vi "Shock&Dyanamics Laboratory - DROPBEAR_June2022_Rev3.vi"() -> ()   [LabVIEW 2019] (continued)
                n641 = property on="Sensitivity 20" class="DigNum (strict)"(error in=w164, "DisabledEnum"=w160) -> (error out=w163:errorcluster)  [unwired: 1 in, 1 out]
                n642 = property on="Sensitivity 19" class="DigNum (strict)"(error in=w173, "DisabledEnum"=w177) -> (error out=w174:errorcluster)  [unwired: 1 in, 1 out]
                n643 = property on="Name Ch 1" class="Str"(error in=w371, "DisabledEnum"=w365) -> (error out=w370:errorcluster)  [unwired: 1 in, 1 out]
                n644 = property on="Physical Channel Ch 27" class="DAQmxName"(error in=w104, "DisabledEnum"=w97) -> (error out=w103:errorcluster)  [unwired: 1 in, 1 out]
                n645 = property on="Name Ch 2" class="Str"(error in=w362, "DisabledEnum"=w356) -> (error out=w361:errorcluster)  [unwired: 1 in, 1 out]
                n646 = property on="Name Ch 4" class="Str"(error in=w346, "DisabledEnum"=w340) -> (error out=w345:errorcluster)  [unwired: 1 in, 1 out]
                n647 = property on="Name Ch 5" class="Str"(error in=w331, "DisabledEnum"=w325) -> (error out=w330:errorcluster)  [unwired: 1 in, 1 out]
                n648 = property on="Name Ch 6" class="Str"(error in=w321, "DisabledEnum"=w315) -> (error out=w320:errorcluster)  [unwired: 1 in, 1 out]
                n649 = property on="Name Ch 12" class="Str"(error in=w262, "DisabledEnum"=w256) -> (error out=w261:errorcluster)  [unwired: 1 in, 1 out]
                n650 = property on="Name Ch 13" class="Str"(error in=w253, "DisabledEnum"=w247) -> (error out=w252:errorcluster)  [unwired: 1 in, 1 out]
                n651 = property on="Name Ch 15" class="Str"(error in=w235, "DisabledEnum"=w229) -> (error out=w234:errorcluster)  [unwired: 1 in, 1 out]
                n652 = property on="Name Ch 7" class="Str"(error in=w312, "DisabledEnum"=w306) -> (error out=w311:errorcluster)  [unwired: 1 in, 1 out]
                n653 = property on="Name Ch 11" class="Str"(error in=w271, "DisabledEnum"=w265) -> (error out=w270:errorcluster)  [unwired: 1 in, 1 out]
                n654 = property on="Name Ch 14" class="Str"(error in=w244, "DisabledEnum"=w238) -> (error out=w243:errorcluster)  [unwired: 1 in, 1 out]
                n655 = property on="Name Ch 8" class="Str"(error in=w301, "DisabledEnum"=w295) -> (error out=w300:errorcluster)  [unwired: 1 in, 1 out]
                n656 = property on="Name Ch 9" class="Str"(error in=w292, "DisabledEnum"=w286) -> (error out=w291:errorcluster)  [unwired: 1 in, 1 out]
                n657 = property on="Name Ch 10" class="Str"(error in=w283, "DisabledEnum"=w277) -> (error out=w282:errorcluster)  [unwired: 1 in, 1 out]
                n658 = property on="Name Ch 16" class="Str"(error in=w220, "DisabledEnum"=w197) -> (error out=w219:errorcluster)  [unwired: 1 in, 1 out]
                n659 = property on="PF Condition 24" class="Bool (strict)"(error in=w130, "DisabledEnum"=w124) -> (error out=w129:errorcluster)  [unwired: 1 in, 1 out]
                n660 = property on="Name Ch 3" class="Str"(error in=w354, "DisabledEnum"=w348) -> (error out=w353:errorcluster)  [unwired: 1 in, 1 out]
                n661 = property on="PF Condition 23" class="Bool (strict)"(error in=w138, "DisabledEnum"=w125) -> (error out=w137:errorcluster)  [unwired: 1 in, 1 out]
                n662 = property on="PF Condition 22" class="Bool (strict)"(error in=w146, "DisabledEnum"=w126) -> (error out=w145:errorcluster)  [unwired: 1 in, 1 out]
                n663 = property on="PF Condition 21" class="Bool (strict)"(error in=w154, "DisabledEnum"=w127) -> (error out=w153:errorcluster)  [unwired: 1 in, 1 out]
                n664 = property on="Sens Fac 17" class="Enum (strict)"(error in=w192, "DisabledEnum"=w187) -> (error out=w188:errorcluster)  [unwired: 1 in, 1 out]
                n665 = property on="PF Condition 20" class="Bool (strict)"(error in=w163, "DisabledEnum"=w160) -> (error out=w162:errorcluster)  [unwired: 1 in, 1 out]
                n666 = property on="PF Condition 19" class="Bool (strict)"(error in=w174, "DisabledEnum"=w177) -> (error out=w175:errorcluster)  [unwired: 1 in, 1 out]
                n667 = property on="PF Condition 18" class="Bool (strict)"(error in=w181, "DisabledEnum"=w178) -> (error out=w180:errorcluster)  [unwired: 1 in, 1 out]
                n668 = property on="Sens Fac 1" class="Enum (strict)"(error in=w370, "DisabledEnum"=w365) -> (error out=w369:errorcluster)  [unwired: 1 in, 1 out]
                n669 = property on="Sens Fac 2" class="Enum (strict)"(error in=w361, "DisabledEnum"=w356) -> (error out=w360:errorcluster)  [unwired: 1 in, 1 out]
                n670 = property on="Name Ch 30" class="Str"(error in=w72, "DisabledEnum"=w78) -> (error out=w73:errorcluster)  [unwired: 1 in, 1 out]
                n671 = property on="Sens Fac 4" class="Enum (strict)"(error in=w345, "DisabledEnum"=w340) -> (error out=w344:errorcluster)  [unwired: 1 in, 1 out]
                n672 = property on="Sens Fac 5" class="Enum (strict)"(error in=w330, "DisabledEnum"=w325) -> (error out=w329:errorcluster)  [unwired: 1 in, 1 out]
                n673 = property on="Sens Fac 6" class="Enum (strict)"(error in=w320, "DisabledEnum"=w315) -> (error out=w319:errorcluster)  [unwired: 1 in, 1 out]
                n674 = property on="Sens Fac 12" class="Enum (strict)"(error in=w261, "DisabledEnum"=w256) -> (error out=w260:errorcluster)  [unwired: 1 in, 1 out]
                n675 = property on="Sens Fac 13" class="Enum (strict)"(error in=w252, "DisabledEnum"=w247) -> (error out=w251:errorcluster)  [unwired: 1 in, 1 out]
                n676 = property on="Sens Fac 15" class="Enum (strict)"(error in=w234, "DisabledEnum"=w229) -> (error out=w233:errorcluster)  [unwired: 1 in, 1 out]
                n677 = property on="Sens Fac 7" class="Enum (strict)"(error in=w311, "DisabledEnum"=w306) -> (error out=w310:errorcluster)  [unwired: 1 in, 1 out]
                n678 = property on="Sens Fac 11" class="Enum (strict)"(error in=w270, "DisabledEnum"=w265) -> (error out=w269:errorcluster)  [unwired: 1 in, 1 out]
                n679 = property on="Sens Fac 14" class="Enum (strict)"(error in=w243, "DisabledEnum"=w238) -> (error out=w242:errorcluster)  [unwired: 1 in, 1 out]
                n680 = property on="Sens Fac 8" class="Enum (strict)"(error in=w300, "DisabledEnum"=w295) -> (error out=w299:errorcluster)  [unwired: 1 in, 1 out]
                n681 = property on="Sens Fac 9" class="Enum (strict)"(error in=w291, "DisabledEnum"=w286) -> (error out=w290:errorcluster)  [unwired: 1 in, 1 out]
                n682 = property on="Sens Fac 10" class="Enum (strict)"(error in=w282, "DisabledEnum"=w277) -> (error out=w281:errorcluster)  [unwired: 1 in, 1 out]
                n683 = property on="Sens Fac 16" class="Enum (strict)"(error in=w219, "DisabledEnum"=w197) -> (error out=w218:errorcluster)  [unwired: 1 in, 1 out]
                n684 = property on="Name Ch 29" class="Str"(error in=w81, "DisabledEnum"=w87) -> (error out=w82:errorcluster)  [unwired: 1 in, 1 out]
                n685 = property on="Name Ch 25" class="Str"(error in=w121, "DisabledEnum"=w115) -> (error out=w120:errorcluster)  [unwired: 1 in, 1 out]
                n686 = property on="Name Ch 26" class="Str"(error in=w108, "DisabledEnum"=w114) -> (error out=w109:errorcluster)  [unwired: 1 in, 1 out]
                n687 = property on="Sens Fac 3" class="Enum (strict)"(error in=w353, "DisabledEnum"=w348) -> (error out=w352:errorcluster)  [unwired: 1 in, 1 out]
                n688 = property on="Name Ch 28" class="Str"(error in=w90, "DisabledEnum"=w96) -> (error out=w91:errorcluster)  [unwired: 1 in, 1 out]
                n689 = property on="Name Ch 27" class="Str"(error in=w103, "DisabledEnum"=w97) -> (error out=w102:errorcluster)  [unwired: 1 in, 1 out]
                n690 = property on="Name Ch 31" class="Str"(error in=w63, "DisabledEnum"=w69) -> (error out=w64:errorcluster)  [unwired: 1 in, 1 out]
                n691 = property on="Sensitivity 17" class="DigNum (strict)"(error in=w188, "DisabledEnum"=w187) -> (error out=w189:errorcluster)  [unwired: 1 in, 1 out]
                n692 = property on="Voltage Min Ch 24" class="DigNum (strict)"(error in=w129, "DisabledEnum"=w124) -> (error out=w128:errorcluster)  [unwired: 1 in, 1 out]
                n693 = property on="Voltage Min Ch 23" class="DigNum (strict)"(error in=w137, "DisabledEnum"=w125) -> (error out=w136:errorcluster)  [unwired: 1 in, 1 out]
                n694 = property on="Sensitivity 1" class="DigNum (strict)"(error in=w369, "DisabledEnum"=w365) -> (error out=w368:errorcluster)  [unwired: 1 in, 1 out]
                n695 = property on="Voltage Min Ch 21" class="DigNum (strict)"(error in=w153, "DisabledEnum"=w127) -> (error out=w152:errorcluster)  [unwired: 1 in, 1 out]
                n696 = property on="Voltage Min Ch 22" class="DigNum (strict)"(error in=w145, "DisabledEnum"=w126) -> (error out=w144:errorcluster)  [unwired: 1 in, 1 out]
                n697 = property on="Voltage Min Ch 20" class="DigNum (strict)"(error in=w162, "DisabledEnum"=w160) -> (error out=w161:errorcluster)  [unwired: 1 in, 1 out]
                n698 = property on="Voltage Min Ch 18" class="DigNum (strict)"(error in=w180, "DisabledEnum"=w178) -> (error out=w179:errorcluster)  [unwired: 1 in, 1 out]
                n699 = property on="Voltage Min Ch 19" class="DigNum (strict)"(error in=w175, "DisabledEnum"=w177) -> (error out=w176:errorcluster)  [unwired: 1 in, 1 out]
                n700 = property on="Sensitivity 2" class="DigNum (strict)"(error in=w360, "DisabledEnum"=w356) -> (error out=w359:errorcluster)  [unwired: 1 in, 1 out]
                n701 = property on="Sensitivity 4" class="DigNum (strict)"(error in=w344, "DisabledEnum"=w340) -> (error out=w343:errorcluster)  [unwired: 1 in, 1 out]
                n702 = property on="Sensitivity 5" class="DigNum (strict)"(error in=w329, "DisabledEnum"=w325) -> (error out=w328:errorcluster)  [unwired: 1 in, 1 out]
                n703 = property on="Sensitivity 6" class="DigNum (strict)"(error in=w319, "DisabledEnum"=w315) -> (error out=w318:errorcluster)  [unwired: 1 in, 1 out]
                n704 = property on="Sensitivity 12" class="DigNum (strict)"(error in=w260, "DisabledEnum"=w256) -> (error out=w259:errorcluster)  [unwired: 1 in, 1 out]
                n705 = property on="Sensitivity 13" class="DigNum (strict)"(error in=w251, "DisabledEnum"=w247) -> (error out=w250:errorcluster)  [unwired: 1 in, 1 out]
                n706 = property on="Sensitivity 15" class="DigNum (strict)"(error in=w233, "DisabledEnum"=w229) -> (error out=w232:errorcluster)  [unwired: 1 in, 1 out]
                n707 = property on="Sensitivity 7" class="DigNum (strict)"(error in=w310, "DisabledEnum"=w306) -> (error out=w309:errorcluster)  [unwired: 1 in, 1 out]
                n708 = property on="Sensitivity 11" class="DigNum (strict)"(error in=w269, "DisabledEnum"=w265) -> (error out=w268:errorcluster)  [unwired: 1 in, 1 out]
                n709 = property on="Sensitivity 14" class="DigNum (strict)"(error in=w242, "DisabledEnum"=w238) -> (error out=w241:errorcluster)  [unwired: 1 in, 1 out]
                n710 = property on="Sensitivity 8" class="DigNum (strict)"(error in=w299, "DisabledEnum"=w295) -> (error out=w298:errorcluster)  [unwired: 1 in, 1 out]
                n711 = property on="Sensitivity 9" class="DigNum (strict)"(error in=w290, "DisabledEnum"=w286) -> (error out=w289:errorcluster)  [unwired: 1 in, 1 out]
                n712 = property on="Sensitivity 10" class="DigNum (strict)"(error in=w281, "DisabledEnum"=w277) -> (error out=w280:errorcluster)  [unwired: 1 in, 1 out]
                n713 = property on="Sensitivity 16" class="DigNum (strict)"(error in=w218, "DisabledEnum"=w197) -> (error out=w217:errorcluster)  [unwired: 1 in, 1 out]
                n714 = property on="Sensitivity 3" class="DigNum (strict)"(error in=w352, "DisabledEnum"=w348) -> (error out=w351:errorcluster)  [unwired: 1 in, 1 out]
                n715 = property on="Sens Fac 30" class="Enum (strict)"(error in=w73, "DisabledEnum"=w78) -> (error out=w74:errorcluster)  [unwired: 1 in, 1 out]
                n716 = property on="Sens Fac 27" class="Enum (strict)"(error in=w102, "DisabledEnum"=w97) -> (error out=w101:errorcluster)  [unwired: 1 in, 1 out]
                n717 = property on="Sens Fac 29" class="Enum (strict)"(error in=w82, "DisabledEnum"=w87) -> (error out=w83:errorcluster)  [unwired: 1 in, 1 out]
                n718 = property on="PF Condition 17" class="Bool (strict)"(error in=w189, "DisabledEnum"=w187) -> (error out=w190:errorcluster)  [unwired: 1 in, 1 out]
                n719 = property on="Sens Fac 26" class="Enum (strict)"(error in=w109, "DisabledEnum"=w114) -> (error out=w110:errorcluster)  [unwired: 1 in, 1 out]
                n720 = property on="Sens Fac 25" class="Enum (strict)"(error in=w120, "DisabledEnum"=w115) -> (error out=w119:errorcluster)  [unwired: 1 in, 1 out]
                n721 = property on="Sens Fac 28" class="Enum (strict)"(error in=w91, "DisabledEnum"=w96) -> (error out=w92:errorcluster)  [unwired: 1 in, 1 out]
                n722 = property on="PF Condition 1" class="Bool (strict)"(error in=w368, "DisabledEnum"=w365) -> (error out=w364:errorcluster)  [unwired: 1 in, 1 out]
                n723 = property on="PF Condition 2" class="Bool (strict)"(error in=w359, "DisabledEnum"=w356) -> (error out=w355:errorcluster)  [unwired: 1 in, 1 out]
                n724 = property on="PF Condition 4" class="Bool (strict)"(error in=w343, "DisabledEnum"=w340) -> (error out=w339:errorcluster)  [unwired: 1 in, 1 out]
                n725 = property on="PF Condition 5" class="Bool (strict)"(error in=w328, "DisabledEnum"=w325) -> (error out=w324:errorcluster)  [unwired: 1 in, 1 out]
                n726 = property on="PF Condition 6" class="Bool (strict)"(error in=w318, "DisabledEnum"=w315) -> (error out=w314:errorcluster)  [unwired: 1 in, 1 out]
                n727 = property on="PF Condition 12" class="Bool (strict)"(error in=w259, "DisabledEnum"=w256) -> (error out=w255:errorcluster)  [unwired: 1 in, 1 out]
                n728 = property on="PF Condition 13" class="Bool (strict)"(error in=w250, "DisabledEnum"=w247) -> (error out=w246:errorcluster)  [unwired: 1 in, 1 out]
                n729 = property on="PF Condition 15" class="Bool (strict)"(error in=w232, "DisabledEnum"=w229) -> (error out=w228:errorcluster)  [unwired: 1 in, 1 out]
                n730 = property on="Sens Fac 31" class="Enum (strict)"(error in=w64, "DisabledEnum"=w69) -> (error out=w65:errorcluster)  [unwired: 1 in, 1 out]
                n731 = property on="PF Condition 7" class="Bool (strict)"(error in=w309, "DisabledEnum"=w306) -> (error out=w305:errorcluster)  [unwired: 1 in, 1 out]
                n732 = property on="PF Condition 11" class="Bool (strict)"(error in=w268, "DisabledEnum"=w265) -> (error out=w264:errorcluster)  [unwired: 1 in, 1 out]
                n733 = property on="PF Condition 14" class="Bool (strict)"(error in=w241, "DisabledEnum"=w238) -> (error out=w237:errorcluster)  [unwired: 1 in, 1 out]
                n734 = property on="PF Condition 8" class="Bool (strict)"(error in=w298, "DisabledEnum"=w295) -> (error out=w294:errorcluster)  [unwired: 1 in, 1 out]
                n735 = property on="PF Condition 9" class="Bool (strict)"(error in=w289, "DisabledEnum"=w286) -> (error out=w285:errorcluster)  [unwired: 1 in, 1 out]
                n736 = property on="PF Condition 10" class="Bool (strict)"(error in=w280, "DisabledEnum"=w277) -> (error out=w276:errorcluster)  [unwired: 1 in, 1 out]
                n737 = property on="Voltage Max Ch 24" class="DigNum (strict)"(error in=w128, "DisabledEnum"=w124) -> ()  [unwired: 1 in, 2 out]
                n738 = property on="PF Condition 16" class="Bool (strict)"(error in=w217, "DisabledEnum"=w197) -> (error out=w215:errorcluster)  [unwired: 1 in, 1 out]
                n739 = property on="Voltage Max Ch 23" class="DigNum (strict)"(error in=w136, "DisabledEnum"=w125) -> ()  [unwired: 1 in, 2 out]
                n740 = property on="Voltage Max Ch 19" class="DigNum (strict)"(error in=w176, "DisabledEnum"=w177) -> ()  [unwired: 1 in, 2 out]
                n741 = property on="Voltage Max Ch 21" class="DigNum (strict)"(error in=w152, "DisabledEnum"=w127) -> ()  [unwired: 1 in, 2 out]
                n742 = property on="Voltage Max Ch 18" class="DigNum (strict)"(error in=w179, "DisabledEnum"=w178) -> ()  [unwired: 1 in, 2 out]
                n743 = property on="PF Condition 3" class="Bool (strict)"(error in=w351, "DisabledEnum"=w348) -> (error out=w347:errorcluster)  [unwired: 1 in, 1 out]
                n744 = property on="Voltage Max Ch 20" class="DigNum (strict)"(error in=w161, "DisabledEnum"=w160) -> ()  [unwired: 1 in, 2 out]
                n745 = property on="Voltage Max Ch 22" class="DigNum (strict)"(error in=w144, "DisabledEnum"=w126) -> ()  [unwired: 1 in, 2 out]
                n746 = property on="Sensitivity 28" class="DigNum (strict)"(error in=w92, "DisabledEnum"=w96) -> (error out=w93:errorcluster)  [unwired: 1 in, 1 out]
                n747 = property on="Sensitivity 30" class="DigNum (strict)"(error in=w74, "DisabledEnum"=w78) -> (error out=w75:errorcluster)  [unwired: 1 in, 1 out]
                n748 = property on="Sensitivity 25" class="DigNum (strict)"(error in=w119, "DisabledEnum"=w115) -> (error out=w118:errorcluster)  [unwired: 1 in, 1 out]
                n749 = property on="Sensitivity 29" class="DigNum (strict)"(error in=w83, "DisabledEnum"=w87) -> (error out=w84:errorcluster)  [unwired: 1 in, 1 out]
                n750 = property on="Sensitivity 26" class="DigNum (strict)"(error in=w110, "DisabledEnum"=w114) -> (error out=w111:errorcluster)  [unwired: 1 in, 1 out]
                n751 = property on="Sensitivity 27" class="DigNum (strict)"(error in=w101, "DisabledEnum"=w97) -> (error out=w100:errorcluster)  [unwired: 1 in, 1 out]
                n752 = property on="Voltage Max Ch 1" class="DigNum (strict)"(error in=w364, "DisabledEnum"=w365) -> (error out=w366:errorcluster)  [unwired: 1 in, 1 out]
                n753 = property on="Voltage Max Ch 17" class="DigNum (strict)"(error in=w190, "DisabledEnum"=w187) -> (error out=w191:errorcluster)  [unwired: 1 in, 1 out]
                n754 = property on="Sensitivity 31" class="DigNum (strict)"(error in=w65, "DisabledEnum"=w69) -> (error out=w66:errorcluster)  [unwired: 1 in, 1 out]
                n755 = property on="Voltage Max Ch 2" class="DigNum (strict)"(error in=w355, "DisabledEnum"=w356) -> (error out=w357:errorcluster)  [unwired: 1 in, 1 out]
                n756 = property on="Voltage Max Ch 4" class="DigNum (strict)"(error in=w339, "DisabledEnum"=w340) -> (error out=w341:errorcluster)  [unwired: 1 in, 1 out]
                n757 = property on="Voltage Max Ch 5" class="DigNum (strict)"(error in=w324, "DisabledEnum"=w325) -> (error out=w326:errorcluster)  [unwired: 1 in, 1 out]
                n758 = property on="Voltage Max  Ch 6" class="DigNum (strict)"(error in=w314, "DisabledEnum"=w315) -> (error out=w316:errorcluster)  [unwired: 1 in, 1 out]
                n759 = property on="Voltage Max Ch 12" class="DigNum (strict)"(error in=w255, "DisabledEnum"=w256) -> (error out=w257:errorcluster)  [unwired: 1 in, 1 out]
                n760 = property on="Voltage Max Ch 13" class="DigNum (strict)"(error in=w246, "DisabledEnum"=w247) -> (error out=w248:errorcluster)  [unwired: 1 in, 1 out]
                n761 = property on="Voltage Max Ch 15" class="DigNum (strict)"(error in=w228, "DisabledEnum"=w229) -> (error out=w230:errorcluster)  [unwired: 1 in, 1 out]
                n762 = property on="Voltage Max Ch 7" class="DigNum (strict)"(error in=w305, "DisabledEnum"=w306) -> (error out=w307:errorcluster)  [unwired: 1 in, 1 out]
                n763 = property on="Voltage Max Ch 11" class="DigNum (strict)"(error in=w264, "DisabledEnum"=w265) -> (error out=w266:errorcluster)  [unwired: 1 in, 1 out]
                n764 = property on="Voltage Max Ch 14" class="DigNum (strict)"(error in=w237, "DisabledEnum"=w238) -> (error out=w239:errorcluster)  [unwired: 1 in, 1 out]
                n765 = property on="Voltage Max Ch 8" class="DigNum (strict)"(error in=w294, "DisabledEnum"=w295) -> (error out=w296:errorcluster)  [unwired: 1 in, 1 out]
                n766 = property on="Voltage Max Ch 9" class="DigNum (strict)"(error in=w285, "DisabledEnum"=w286) -> (error out=w287:errorcluster)  [unwired: 1 in, 1 out]
                n767 = property on="Voltage Max Ch 10" class="DigNum (strict)"(error in=w276, "DisabledEnum"=w277) -> (error out=w278:errorcluster)  [unwired: 1 in, 1 out]
                n768 = property on="Voltage Max Ch 16" class="DigNum (strict)"(error in=w215, "DisabledEnum"=w197) -> (error out=w216:errorcluster)  [unwired: 1 in, 1 out]
                n769 = property on="Voltage Max Ch 3" class="DigNum (strict)"(error in=w347, "DisabledEnum"=w348) -> (error out=w349:errorcluster)  [unwired: 1 in, 1 out]
                n770 = property on="PF Condition 28" class="Bool (strict)"(error in=w93, "DisabledEnum"=w96) -> (error out=w94:errorcluster)  [unwired: 1 in, 1 out]
                n771 = property on="PF Condition 30" class="Bool (strict)"(error in=w75, "DisabledEnum"=w78) -> (error out=w76:errorcluster)  [unwired: 1 in, 1 out]
                n772 = property on="PF Condition 29" class="Bool (strict)"(error in=w84, "DisabledEnum"=w87) -> (error out=w85:errorcluster)  [unwired: 1 in, 1 out]
                n773 = property on="PF Condition 25" class="Bool (strict)"(error in=w118, "DisabledEnum"=w115) -> (error out=w117:errorcluster)  [unwired: 1 in, 1 out]
                n774 = property on="PF Condition 27" class="Bool (strict)"(error in=w100, "DisabledEnum"=w97) -> (error out=w99:errorcluster)  [unwired: 1 in, 1 out]
                n775 = property on="PF Condition 26" class="Bool (strict)"(error in=w111, "DisabledEnum"=w114) -> (error out=w112:errorcluster)  [unwired: 1 in, 1 out]
                n776 = property on="PF Condition 31" class="Bool (strict)"(error in=w66, "DisabledEnum"=w69) -> (error out=w67:errorcluster)  [unwired: 1 in, 1 out]
                n777 = property on="Voltage Min Ch 1" class="DigNum (strict)"(error in=w366, "DisabledEnum"=w365) -> ()  [unwired: 1 in, 2 out]
                n778 = property on="Voltage Min Ch 17" class="DigNum (strict)"(error in=w191, "DisabledEnum"=w187) -> ()  [unwired: 1 in, 2 out]
                n779 = property on="Voltage Min Ch 2" class="DigNum (strict)"(error in=w357, "DisabledEnum"=w356) -> ()  [unwired: 1 in, 2 out]
                n780 = property on="Voltage Min Ch 4" class="DigNum (strict)"(error in=w341, "DisabledEnum"=w340) -> ()  [unwired: 1 in, 2 out]
                n781 = property on="Voltage Min Ch 5" class="DigNum (strict)"(error in=w326, "DisabledEnum"=w325) -> ()  [unwired: 1 in, 2 out]
                n782 = property on="Voltage Min Ch 6" class="DigNum (strict)"(error in=w316, "DisabledEnum"=w315) -> ()  [unwired: 1 in, 2 out]
                n783 = property on="Voltage Min Ch 12" class="DigNum (strict)"(error in=w257, "DisabledEnum"=w256) -> ()  [unwired: 1 in, 2 out]
                n784 = property on="Voltage Min Ch 13" class="DigNum (strict)"(error in=w248, "DisabledEnum"=w247) -> ()  [unwired: 1 in, 2 out]
                n785 = property on="Voltage Min Ch 15" class="DigNum (strict)"(error in=w230, "DisabledEnum"=w229) -> ()  [unwired: 1 in, 2 out]
                n786 = property on="Voltage Min Ch 7" class="DigNum (strict)"(error in=w307, "DisabledEnum"=w306) -> ()  [unwired: 1 in, 2 out]
                n787 = property on="Voltage Min Ch 11" class="DigNum (strict)"(error in=w266, "DisabledEnum"=w265) -> ()  [unwired: 1 in, 2 out]
                n788 = property on="Voltage Min Ch 14" class="DigNum (strict)"(error in=w239, "DisabledEnum"=w238) -> ()  [unwired: 1 in, 2 out]
                n789 = property on="Voltage Min Ch 8" class="DigNum (strict)"(error in=w296, "DisabledEnum"=w295) -> ()  [unwired: 1 in, 2 out]
                n790 = property on="Voltage Min Ch 9" class="DigNum (strict)"(error in=w287, "DisabledEnum"=w286) -> ()  [unwired: 1 in, 2 out]
                n791 = property on="Voltage Min Ch 10" class="DigNum (strict)"(error in=w278, "DisabledEnum"=w277) -> ()  [unwired: 1 in, 2 out]
                n792 = property on="Voltage Min Ch 16" class="DigNum (strict)"(error in=w216, "DisabledEnum"=w197) -> ()  [unwired: 1 in, 2 out]
                n793 = property on="Voltage Min Ch 3" class="DigNum (strict)"(error in=w349, "DisabledEnum"=w348) -> ()  [unwired: 1 in, 2 out]
                n794 = property on="Voltage Min Ch 30" class="DigNum (strict)"(error in=w76, "DisabledEnum"=w78) -> (error out=w77:errorcluster)  [unwired: 1 in, 1 out]
                n795 = property on="Voltage Min Ch 28" class="DigNum (strict)"(error in=w94, "DisabledEnum"=w96) -> (error out=w95:errorcluster)  [unwired: 1 in, 1 out]
                n796 = property on="Voltage Min Ch 29" class="DigNum (strict)"(error in=w85, "DisabledEnum"=w87) -> (error out=w86:errorcluster)  [unwired: 1 in, 1 out]
                n797 = property on="Voltage Min Ch 27" class="DigNum (strict)"(error in=w99, "DisabledEnum"=w97) -> (error out=w98:errorcluster)  [unwired: 1 in, 1 out]
                n798 = property on="Voltage Min Ch 25" class="DigNum (strict)"(error in=w117, "DisabledEnum"=w115) -> (error out=w116:errorcluster)  [unwired: 1 in, 1 out]
                n799 = property on="Voltage Min Ch 31" class="DigNum (strict)"(error in=w67, "DisabledEnum"=w69) -> (error out=w68:errorcluster)  [unwired: 1 in, 1 out]
                n800 = property on="Voltage Min Ch 26" class="DigNum (strict)"(error in=w112, "DisabledEnum"=w114) -> (error out=w113:errorcluster)  [unwired: 1 in, 1 out]
                n801 = property on="Voltage Max Ch 30" class="DigNum (strict)"(error in=w77, "DisabledEnum"=w78) -> ()  [unwired: 1 in, 2 out]
                n802 = property on="Voltage Max Ch 25" class="DigNum (strict)"(error in=w116, "DisabledEnum"=w115) -> ()  [unwired: 1 in, 2 out]
                n803 = property on="Voltage Max Ch 29" class="DigNum (strict)"(error in=w86, "DisabledEnum"=w87) -> ()  [unwired: 1 in, 2 out]
                n804 = property on="Voltage Max Ch 28" class="DigNum (strict)"(error in=w95, "DisabledEnum"=w96) -> ()  [unwired: 1 in, 2 out]
                n805 = property on="Voltage Max Ch 27" class="DigNum (strict)"(error in=w98, "DisabledEnum"=w97) -> ()  [unwired: 1 in, 2 out]
                n806 = property on="Voltage Max Ch 31" class="DigNum (strict)"(error in=w68, "DisabledEnum"=w69) -> ()  [unwired: 1 in, 2 out]
                n807 = property on="Voltage Max Ch 26" class="DigNum (strict)"(error in=w113, "DisabledEnum"=w114) -> ()  [unwired: 1 in, 2 out]
              }
              event "SG Pair 0", "SG Pair 1", "SG Pair 2", "SG Pair 3", "SG Pair 4", "SG Pair 5", "SG Pair 6", "SG Pair 7", "SG Pair 8", "SG Pair 9", "SG Pair 10", "SG Pair 11", "SG Pair 12", "SG Pair 13", "SG Pair 14", "SG Pair 15", "SG Pair 16", "SG Pair 17", "SG Pair 18", "SG Pair 19", "SG Pair 20", "SG Pair 21", "SG Pair 22", "SG Pair 23", "SG Pair 24", "SG Pair 25", "SG Pair 26", "SG Pair 27", "SG Pair 28", "SG Pair 29", "SG Pair 30", "SG Pair 31": Value Change {
                n808 = event-data() -> ()  [unwired: 1 in, 5 out]
                n809 = property on="SG Pair 30" class="Bool (strict)"() -> ("Value"=w1099:bool)  [unwired: 2 in, 2 out]
                n810 = property on="SG Pair 25" class="Bool (strict)"() -> ("Value"=w1094:bool)  [unwired: 2 in, 2 out]
                n811 = property on="SG Pair 26" class="Bool (strict)"() -> ("Value"=w1095:bool)  [unwired: 2 in, 2 out]
                n812 = property on="SG Pair 28" class="Bool (strict)"() -> ("Value"=w1097:bool)  [unwired: 2 in, 2 out]
                n813 = property on="SG Pair 29" class="Bool (strict)"() -> ("Value"=w1098:bool)  [unwired: 2 in, 2 out]
                n814 = property on="SG Pair 24" class="Bool (strict)"() -> ("Value"=w1093:bool)  [unwired: 2 in, 2 out]
                n815 = property on="SG Pair 27" class="Bool (strict)"() -> ("Value"=w1096:bool)  [unwired: 2 in, 2 out]
                n816 = property on="SG Pair 22" class="Bool (strict)"() -> ("Value"=w1091:bool)  [unwired: 2 in, 2 out]
                n817 = property on="SG Pair 31" class="Bool (strict)"() -> ("Value"=w1100:bool)  [unwired: 2 in, 2 out]
                n818 = property on="SG Pair 21" class="Bool (strict)"() -> ("Value"=w1090:bool)  [unwired: 2 in, 2 out]
                n819 = property on="SG Pair 23" class="Bool (strict)"() -> ("Value"=w1092:bool)  [unwired: 2 in, 2 out]
                n820 = property on="SG Pair 19" class="Bool (strict)"() -> ("Value"=w1088:bool)  [unwired: 2 in, 2 out]
                n821 = property on="SG Pair 18" class="Bool (strict)"() -> ("Value"=w1087:bool)  [unwired: 2 in, 2 out]
                n822 = property on="SG Pair 20" class="Bool (strict)"() -> ("Value"=w1089:bool)  [unwired: 2 in, 2 out]
                n823 = property on="SG Pair 0" class="Bool (strict)"() -> ("Value"=w1119:bool)  [unwired: 2 in, 2 out]
                n824 = property on="SG Pair 1" class="Bool (strict)"() -> ("Value"=w1118:bool)  [unwired: 2 in, 2 out]
                n825 = property on="SG Pair 2" class="Bool (strict)"() -> ("Value"=w1117:bool)  [unwired: 2 in, 2 out]
                n826 = property on="SG Pair 3" class="Bool (strict)"() -> ("Value"=w1116:bool)  [unwired: 2 in, 2 out]
                n827 = property on="SG Pair 4" class="Bool (strict)"() -> ("Value"=w1115:bool)  [unwired: 2 in, 2 out]
                n828 = property on="SG Pair 5" class="Bool (strict)"() -> ("Value"=w1114:bool)  [unwired: 2 in, 2 out]
                n829 = property on="SG Pair 6" class="Bool (strict)"() -> ("Value"=w1113:bool)  [unwired: 2 in, 2 out]
                n830 = property on="SG Pair 7" class="Bool (strict)"() -> ("Value"=w1112:bool)  [unwired: 2 in, 2 out]
                n831 = property on="SG Pair 8" class="Bool (strict)"() -> ("Value"=w1111:bool)  [unwired: 2 in, 2 out]
                n832 = property on="SG Pair 9" class="Bool (strict)"() -> ("Value"=w1110:bool)  [unwired: 2 in, 2 out]
                n833 = property on="SG Pair 10" class="Bool (strict)"() -> ("Value"=w1109:bool)  [unwired: 2 in, 2 out]
                n834 = property on="SG Pair 11" class="Bool (strict)"() -> ("Value"=w1108:bool)  [unwired: 2 in, 2 out]
                n835 = property on="SG Pair 12" class="Bool (strict)"() -> ("Value"=w1107:bool)  [unwired: 2 in, 2 out]
                n836 = property on="SG Pair 13" class="Bool (strict)"() -> ("Value"=w1106:bool)  [unwired: 2 in, 2 out]
                n837 = property on="SG Pair 14" class="Bool (strict)"() -> ("Value"=w1105:bool)  [unwired: 2 in, 2 out]
                n838 = property on="SG Pair 15" class="Bool (strict)"() -> ("Value"=w1104:bool)  [unwired: 2 in, 2 out]
                n839 = property on="SG Pair 16" class="Bool (strict)"() -> ("Value"=w1102:bool)  [unwired: 2 in, 2 out]
                n840 = property on="SG Pair 17" class="Bool (strict)"() -> ("Value"=w1101:bool)  [unwired: 2 in, 2 out]
                n841 = case shown="True" w1119 {
                  tunnel: [T42."Disabled and Grayed Out" ("Disabled") T42."Enabled" ("Disabled")] -> w1086
                  frame False {
                  }
                  frame True {
                  }
                }
                n842 = case shown="True" w1118 {
                  tunnel: [T42."Disabled and Grayed Out" ("Disabled") T42."Enabled" ("Disabled")] -> w1085
                  frame False {
                  }
                  frame True {
                  }
                }
                n843 = case shown="True" w1117 {
                  tunnel: [T42."Disabled and Grayed Out" ("Disabled") T42."Enabled" ("Disabled")] -> w1084
                  frame False {
                  }
                  frame True {
                  }
                }
                n844 = case shown="True" w1116 {
                  tunnel: [T42."Disabled and Grayed Out" ("Disabled") T42."Enabled" ("Disabled")] -> w1083
                  frame False {
                  }
                  frame True {
                  }
                }
                n845 = case shown="True" w1115 {
                  tunnel: [T42."Disabled and Grayed Out" ("Disabled") T42."Enabled" ("Disabled")] -> w1082
                  frame False {
                  }
                  frame True {
                  }
                }
                n846 = case shown="True" w1114 {
                  tunnel: [T42."Disabled and Grayed Out" ("Disabled") T42."Enabled" ("Disabled")] -> w1081
                  frame False {
                  }
                  frame True {
                  }
                }
                n847 = case shown="True" w1113 {
                  tunnel: [T42."Disabled and Grayed Out" ("Disabled") T42."Enabled" ("Disabled")] -> w1080
                  frame False {
                  }
                  frame True {
                  }
                }
                n848 = case shown="True" w1112 {
                  tunnel: [T42."Disabled and Grayed Out" ("Disabled") T42."Enabled" ("Disabled")] -> w1079
                  frame False {
                  }
                  frame True {
                  }
                }
                n849 = case shown="True" w1111 {
                  tunnel: [T42."Disabled and Grayed Out" ("Disabled") T42."Enabled" ("Disabled")] -> w1078
                  frame False {
                  }
                  frame True {
                  }
                }
                n850 = case shown="True" w1110 {
                  tunnel: [T42."Disabled and Grayed Out" ("Disabled") T42."Enabled" ("Disabled")] -> w1077
                  frame False {
                  }
                  frame True {
                  }
                }
                n851 = case shown="True" w1109 {
                  tunnel: [T42."Disabled and Grayed Out" ("Disabled") T42."Enabled" ("Disabled")] -> w1076
                  frame False {
                  }
                  frame True {
                  }
                }
                n852 = case shown="True" w1108 {
                  tunnel: [T42."Disabled and Grayed Out" ("Disabled") T42."Enabled" ("Disabled")] -> w1075
                  frame False {
                  }
                  frame True {
                  }
                }
                n853 = case shown="True" w1107 {
                  tunnel: [T42."Disabled and Grayed Out" ("Disabled") T42."Enabled" ("Disabled")] -> w1074
                  frame False {
                  }
                  frame True {
                  }
                }
                n854 = case shown="True" w1106 {
                  tunnel: [T42."Disabled and Grayed Out" ("Disabled") T42."Enabled" ("Disabled")] -> w1073
                  frame False {
                  }
                  frame True {
                  }
                }
                n855 = case shown="True" w1105 {
                  tunnel: [T42."Disabled and Grayed Out" ("Disabled") T42."Enabled" ("Disabled")] -> w1067
                  frame False {
                  }
                  frame True {
                  }
                }
                n856 = case shown="True" w1104 {
                  tunnel: [T42."Disabled and Grayed Out" ("Disabled") T42."Enabled" ("Disabled")] -> w1068
                  frame False {
                  }
                  frame True {
                  }
                }
                n857 = case shown="True" w1102 {
                  tunnel: [T42."Disabled and Grayed Out" ("Disabled") T42."Enabled" ("Disabled")] -> w1072
                  frame False {
                  }
                  frame True {
                  }
                }
                n858 = case shown="True" w1101 {
                  tunnel: [T42."Disabled and Grayed Out" ("Disabled") T42."Enabled" ("Disabled")] -> w1071
                  frame False {
                  }
                  frame True {
                  }
                }
                n859 = case shown="True" w1087 {
                  tunnel: [T42."Disabled and Grayed Out" ("Disabled") T42."Enabled" ("Disabled")] -> w1070
                  frame False {
                  }
                  frame True {
                  }
                }
                n860 = case shown="True" w1088 {
                  tunnel: [T42."Disabled and Grayed Out" ("Disabled") T42."Enabled" ("Disabled")] -> w1069
                  frame False {
                  }
                  frame True {
                  }
                }
                n861 = case shown="True" w1089 {
                  tunnel: [T42."Disabled and Grayed Out" ("Disabled") T42."Enabled" ("Disabled")] -> w1055
                  frame False {
                  }
                  frame True {
                  }
                }
                n862 = case shown="True" w1090 {
                  tunnel: [T42."Disabled and Grayed Out" ("Disabled") T42."Enabled" ("Disabled")] -> w1056
                  frame False {
                  }
                  frame True {
                  }
                }
                n863 = case shown="True" w1091 {
                  tunnel: [T42."Disabled and Grayed Out" ("Disabled") T42."Enabled" ("Disabled")] -> w1057
                  frame False {
                  }
                  frame True {
                  }
                }
                n864 = case shown="True" w1092 {
                  tunnel: [T42."Disabled and Grayed Out" ("Disabled") T42."Enabled" ("Disabled")] -> w1058
                  frame False {
                  }
                  frame True {
                  }
                }
                n865 = case shown="True" w1093 {
                  tunnel: [T42."Disabled and Grayed Out" ("Disabled") T42."Enabled" ("Disabled")] -> w1059
                  frame False {
                  }
                  frame True {
                  }
                }
                n866 = case shown="True" w1094 {
                  tunnel: [T42."Disabled and Grayed Out" ("Disabled") T42."Enabled" ("Disabled")] -> w1060
                  frame False {
                  }
                  frame True {
                  }
                }
                n867 = case shown="True" w1095 {
                  tunnel: [T42."Disabled and Grayed Out" ("Disabled") T42."Enabled" ("Disabled")] -> w1061
                  frame False {
                  }
                  frame True {
                  }
                }
                n868 = case shown="True" w1096 {
                  tunnel: [T42."Disabled and Grayed Out" ("Disabled") T42."Enabled" ("Disabled")] -> w1062
                  frame False {
                  }
                  frame True {
                  }
                }
                n869 = case shown="True" w1097 {
                  tunnel: [T42."Disabled and Grayed Out" ("Disabled") T42."Enabled" ("Disabled")] -> w1063
                  frame False {
                  }
                  frame True {
                  }
                }
                n870 = case shown="True" w1098 {
                  tunnel: [T42."Disabled and Grayed Out" ("Disabled") T42."Enabled" ("Disabled")] -> w1064
                  frame False {
                  }
                  frame True {
                  }
                }
                n871 = case shown="True" w1099 {
                  tunnel: [T42."Disabled and Grayed Out" ("Disabled") T42."Enabled" ("Disabled")] -> w1065
                  frame False {
                  }
                  frame True {
                  }
                }
                n872 = case shown="True" w1100 {
                  tunnel: [T42."Disabled and Grayed Out" ("Disabled") T42."Enabled" ("Disabled")] -> w1066
                  frame False {
                  }
                  frame True {
                  }
                }
                n873 = property on="SG Pair Ch 2" class="Enum (strict)"("DisabledEnum"=w1084) -> ()  [unwired: 2 in, 2 out]
                n874 = property on="SG Pair Ch 0" class="Enum (strict)"("DisabledEnum"=w1086) -> ()  [unwired: 2 in, 2 out]
                n875 = property on="SG Pair Ch 3" class="Enum (strict)"("DisabledEnum"=w1083) -> ()  [unwired: 2 in, 2 out]
                n876 = property on="SG Pair Ch 1" class="Enum (strict)"("DisabledEnum"=w1085) -> ()  [unwired: 2 in, 2 out]
                n877 = property on="SG Pair Ch 13" class="Enum (strict)"("DisabledEnum"=w1073) -> ()  [unwired: 2 in, 2 out]
                n878 = property on="SG Pair Ch 12" class="Enum (strict)"("DisabledEnum"=w1074) -> ()  [unwired: 2 in, 2 out]
                n879 = property on="SG Pair Ch 10" class="Enum (strict)"("DisabledEnum"=w1076) -> ()  [unwired: 2 in, 2 out]
                n880 = property on="SG Pair Ch 8" class="Enum (strict)"("DisabledEnum"=w1078) -> ()  [unwired: 2 in, 2 out]
                n881 = property on="SG Pair Ch 11" class="Enum (strict)"("DisabledEnum"=w1075) -> ()  [unwired: 2 in, 2 out]
                n882 = property on="SG Pair Ch 9" class="Enum (strict)"("DisabledEnum"=w1077) -> ()  [unwired: 2 in, 2 out]
                n883 = property on="SG Pair Ch 14" class="Enum (strict)"("DisabledEnum"=w1067) -> ()  [unwired: 2 in, 2 out]
                n884 = property on="SG Pair Ch 15" class="Enum (strict)"("DisabledEnum"=w1068) -> ()  [unwired: 2 in, 2 out]
                n885 = property on="SG Pair Ch 6" class="Enum (strict)"("DisabledEnum"=w1080) -> ()  [unwired: 2 in, 2 out]
                n886 = property on="SG Pair Ch 4" class="Enum (strict)"("DisabledEnum"=w1082) -> ()  [unwired: 2 in, 2 out]
                n887 = property on="SG Pair Ch 7" class="Enum (strict)"("DisabledEnum"=w1079) -> ()  [unwired: 2 in, 2 out]
                n888 = property on="SG Pair Ch 5" class="Enum (strict)"("DisabledEnum"=w1081) -> ()  [unwired: 2 in, 2 out]
